vi "imagein.vi"() -> ()   [LabVIEW 2012]
panel:
  out "remote address":string caption="远程地址"
  out "错误输出":errorcluster
  out "x+y":u32
  in  "停止":bool
  out "*(类型 *) &x":i32
  out "添加的路径":path
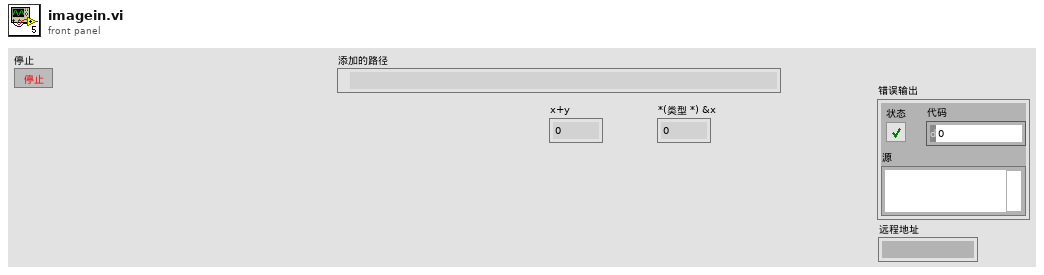
[diagram p1: front panel]
types:
  T1 = enum16{"open", "replace", "create", "open or create", "replace or create", "replace or create with confirmation"}
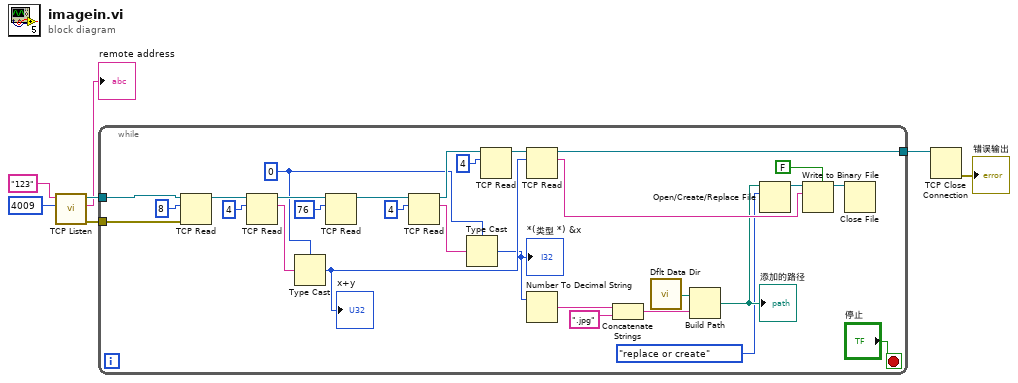
[diagram p0: block diagram]
diagram:
  n1 = call <vilib>:"TCP Listen.vi"("port"=u16 4009, "service name"="123") -> ("error out"=w5:errorcluster, "remote address"=→"remote address":string, "connection ID"=w6:refnum<k5>)  [unwired: 5 in, 2 out]
  n2 = while {
    tunnel: w6 -> [w36]
    tunnel: w5 -> [w34]
    tunnel: [w23] -> w1
    stop <- "停止" stop-if-true
    w20 = 0
    n3 = TCP Read(connection ID=w36, bytes to read=8 ("读取的字节"), error in (no error)=w34) -> (connection ID out=w33:refnum<k5>)  [unwired: 2 in, 2 out]
    n4 = TCP Read(connection ID=w33, bytes to read=4 ("读取的字节")) -> (connection ID out=w30:refnum<k5>, data out=w21:string)  [unwired: 3 in, 1 out]
    n5 = Type Cast(type=w20, x=w21) -> (*(type *) &x=w17:i32)
    "x+y" <- w17
    n6 = TCP Read(connection ID=w30, bytes to read=76 ("读取的字节")) -> (connection ID out=w28:refnum<k5>)  [unwired: 3 in, 2 out]
    n7 = TCP Read(connection ID=w28, bytes to read=4 ("读取的字节")) -> (connection ID out=w26:refnum<k5>, data out=w22:string)  [unwired: 3 in, 1 out]
    n8 = Type Cast(type=w20, x=w22) -> (*(type *) &x=w13:i32)
    "*(类型 *) &x" <- w13
    n9 = TCP Read(connection ID=w26, bytes to read=4 ("读取的字节")) -> (connection ID out=w24:refnum<k5>)  [unwired: 3 in, 2 out]
    n10 = TCP Read(connection ID=w24, bytes to read=w17) -> (connection ID out=w23:refnum<k5>, data out=w15:string)  [unwired: 3 in, 1 out]
    n11 = Number To Decimal String(number=w13) -> (decimal integer string=w12:string)  [unwired: 1 in]
    n12 = Concatenate Strings(w12, ".jpg" ("字符串")) -> (w10:string)
    n13 = call <vilib>:"Dflt Data Dir.vi"() -> ("App:Default Data Directory"=w14:path)
    n14 = Build Path(base path=w14, name or relative path=w10) -> (appended path=w9:path)
    "添加的路径" <- w9
    n15 = Open/Create/Replace File(file path (use dialog)=w9, operation (0:open)=T1."replace or create" ("操作(0:open)")) -> (refnum out=w18:refnum<file>)  [unwired: 4 in, 2 out]
    n16 = Write to Binary File(file (use dialog)=w18, data=w15, 5:FALSE ("预置数组或字符串大小？(T)")) -> (refnum out=w19:refnum<file>)  [unwired: 3 in, 2 out]
    n17 = Close File(refnum=w19) -> ()  [unwired: 1 in, 2 out]
  }
  n18 = TCP Close Connection(connection ID=w1) -> (error out=→"错误输出":errorcluster)  [unwired: 2 in, 1 out]
